vi "Event Tree.vi"   [LabVIEW 2013]
uses:
  <resource>/importtools/Common/Event/NISAST Event.lvclass
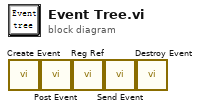
[diagram p0: block diagram]
diagram:
  n1 = call-dynamic "Create Event.vi"() -> ()  [unwired: 9 in, 3 out]
  n2 = call-dynamic "Post Event.vi"() -> ()  [unwired: 10 in, 2 out]
  n3 = call-dynamic "Reg Ref.vi"() -> ()  [unwired: 9 in, 3 out]
  n4 = call-dynamic "Send Event.vi"() -> ()  [unwired: 9 in, 3 out]
  n5 = call-dynamic "Destroy Event.vi"() -> ()  [unwired: 10 in, 2 out]
